vi "TreeItem.Property.Get.vi"(6 "Custom Device Path":string, 8 "error in (no error)":errorcluster, 9 "Default Value":variant, 10 "Property Name":string, 11 "Basenode":refnum<k24>) -> (0 "error out":errorcluster, 1 "Variant":variant, 2 "Found?":bool, 3 "Basenode":refnum<k24>)   [LabVIEW 2016, in "Advanced System Definition.lvlib"]
uses:
  SysDef API/Advanced System Definition.lvlib
  NationalInstruments.VeriStand.SystemStorage
  _Types/Property.DependentFile.ctl
  NationalInstruments.VeriStand
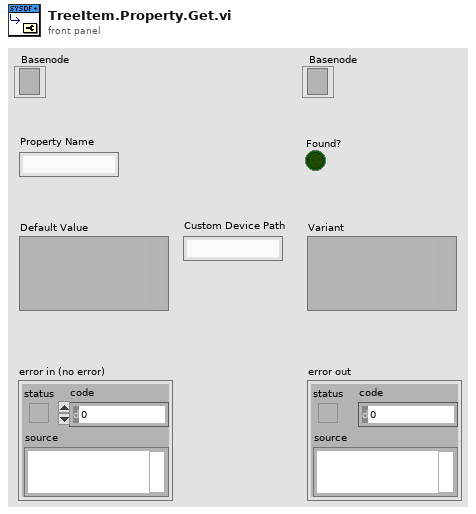
[diagram p1: front panel]
types:
  T1 = typedef "Advanced System Definition.lvlib/Property.DependentFile.ctl" = cluster{"Original Path":path, "Version":string, "RTDestination":path, "ForceDownload":bool, "SupportedTarget":string, "MD5":string}
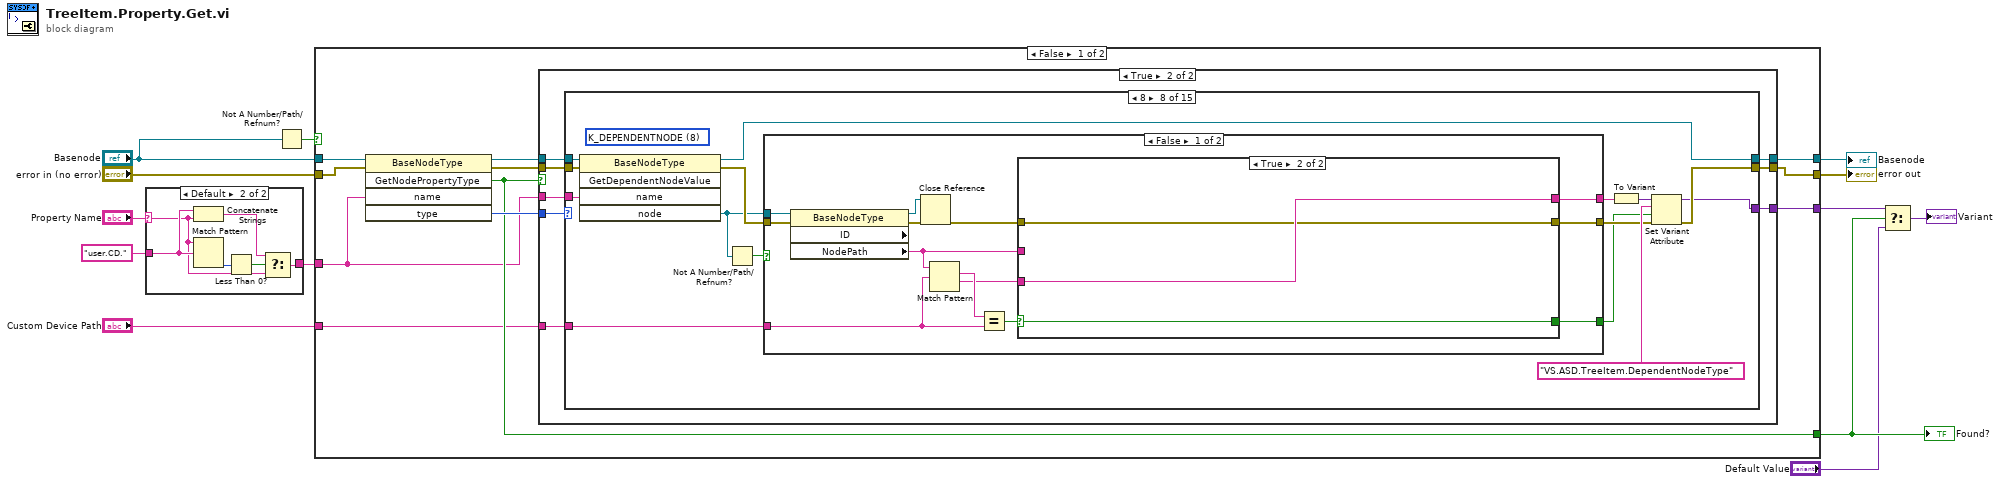
[diagram p0: block diagram]
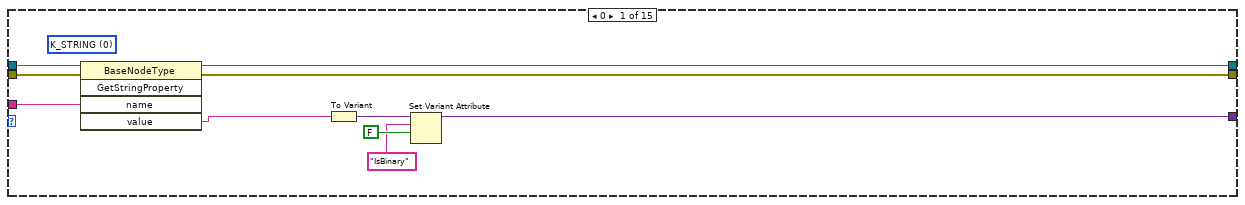
[diagram p4: hidden frame]
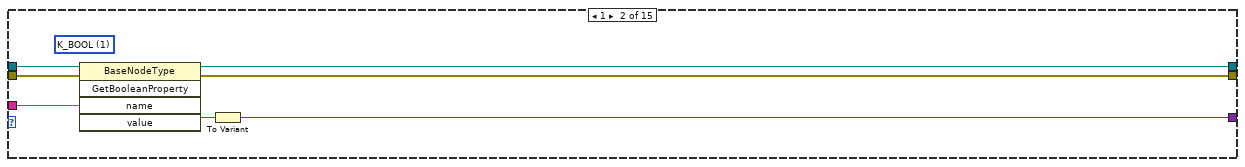
[diagram p5: hidden frame]
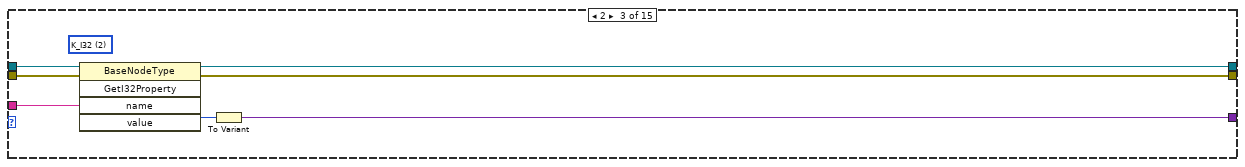
[diagram p6: hidden frame]
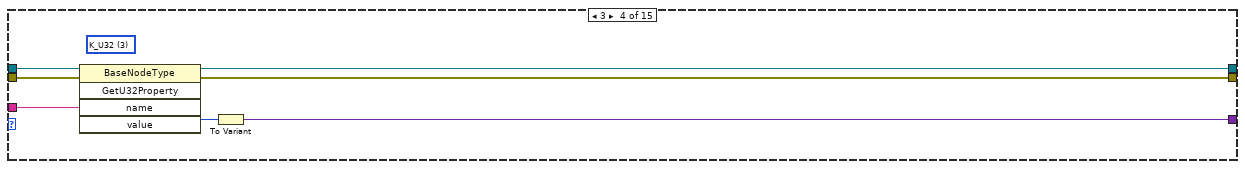
[diagram p7: hidden frame]
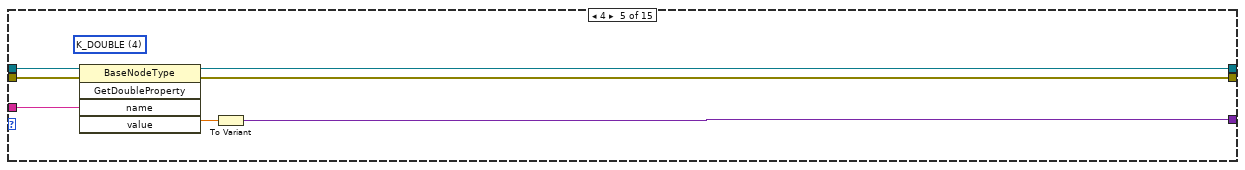
[diagram p8: hidden frame]
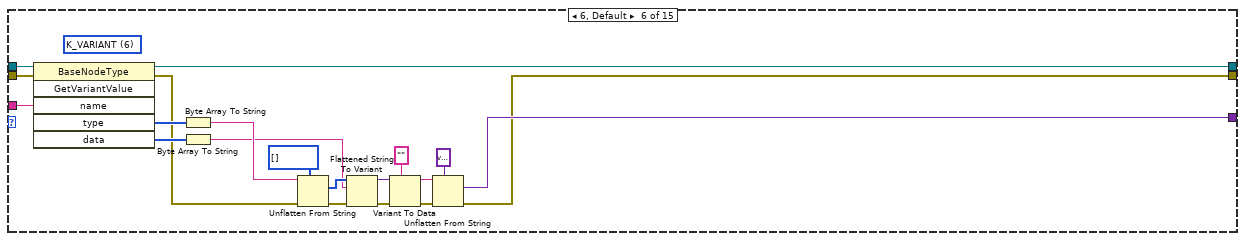
[diagram p9: hidden frame]
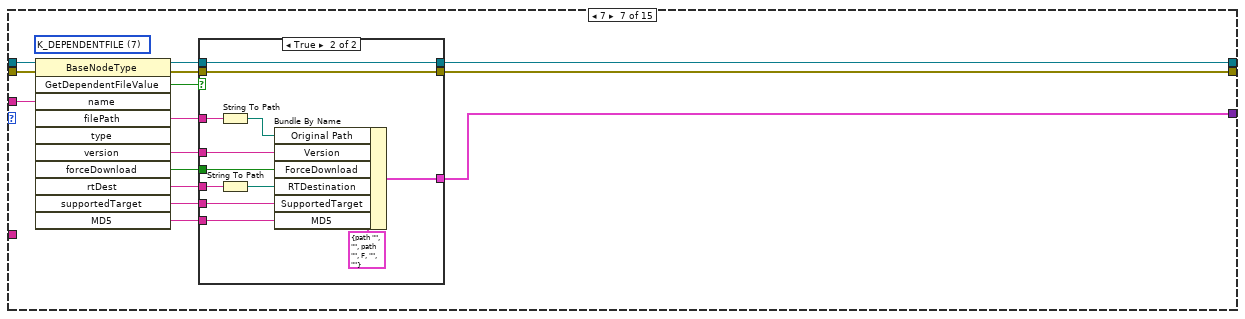
[diagram p10: hidden frame]
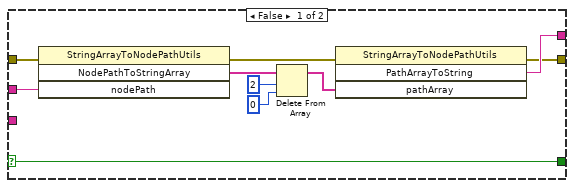
[diagram p12: hidden frame]
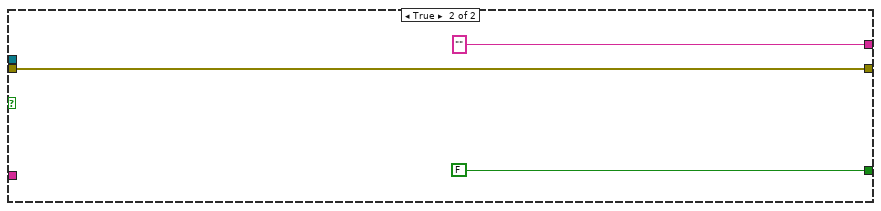
[diagram p13: hidden frame]
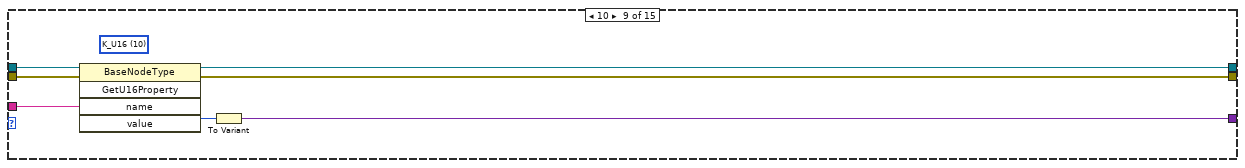
[diagram p14: hidden frame]
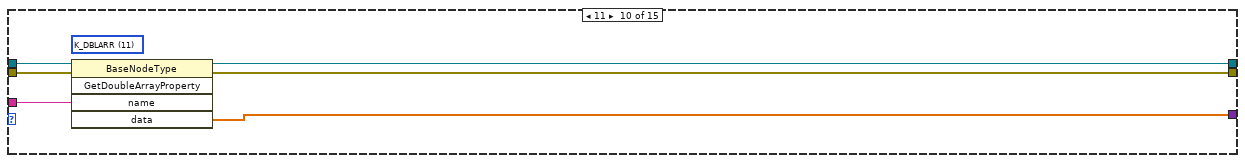
[diagram p15: hidden frame]
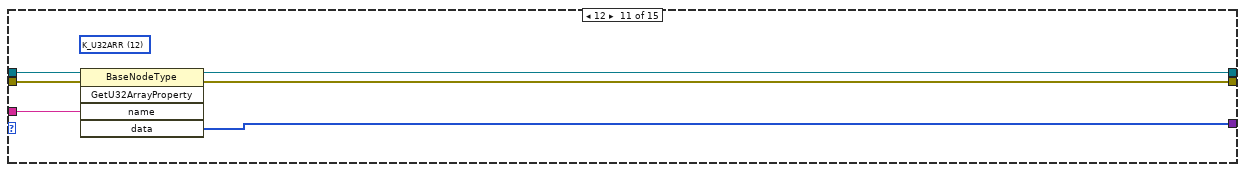
[diagram p16: hidden frame]
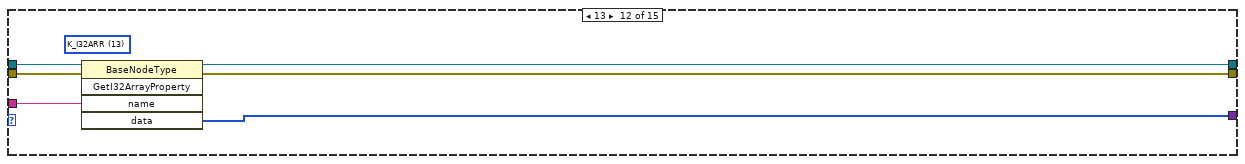
[diagram p17: hidden frame]
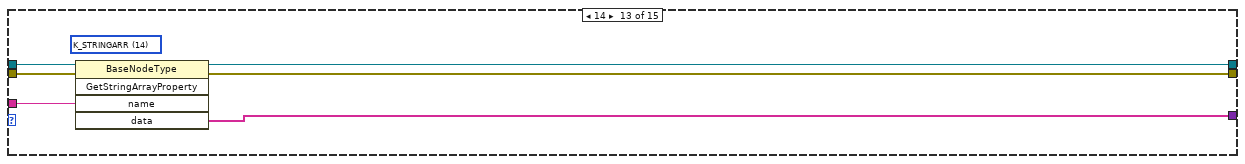
[diagram p18: hidden frame]
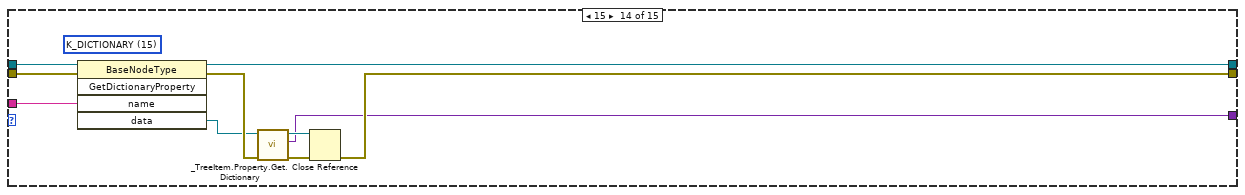
[diagram p19: hidden frame]
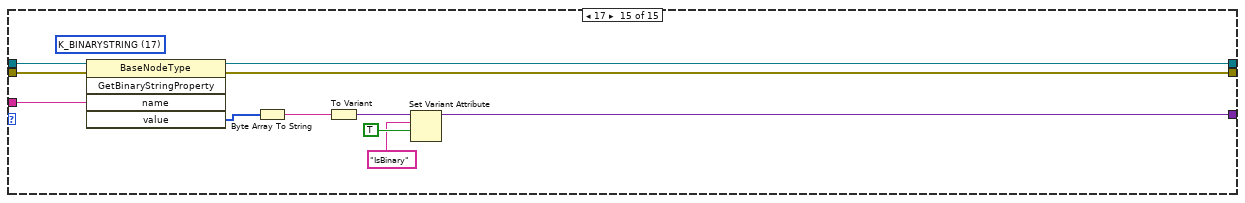
[diagram p20: hidden frame]
diagram:
  n1 = case shown="Default" "Property Name" {
    selector: "Property Name" -> [w14 w15]
    tunnel: "user.CD." ("regular expression") -> [_ w18]
    tunnel: [w14 w16] -> w3
    frame "Value Table" {
    }
    frame Default {
      n2 = Concatenate Strings(w18, w15) -> (w19:string)
      n3 = Match Pattern(string=w15, regular expression=w18) -> (offset past match=w20:i32)  [unwired: 1 in, 3 out]
      n4 = Less Than 0?(x=w20) -> (x < 0?=w17:bool)
      n5 = Select(t=w19, s=w17, f=w15) -> (s? t:f=w16:string)
    }
  }
  n6 = Not A Number/Path/Refnum?(number/path/refnum="Basenode") -> (NaN/Path/Refnum?=w13:bool)
  n7 = case shown="False" w13 {
    tunnel: w3 -> [w22 _]
    tunnel: "Basenode" -> [w31 w226]
    tunnel: "error in (no error)" -> [w30 w225]
    tunnel: [w26 _] -> w10
    tunnel: [w25 _] -> w9
    tunnel: [w24 w226] -> w6
    tunnel: [w23 w225] -> w5
    tunnel: "Custom Device Path" -> [w21 _]
    frame False {
      n8 = invoke class="BaseNodeType" method="GetNodePropertyType"(reference=w31, error in=w30, "name"=w22) -> (reference out=w27:refnum<k24>, error out=w29:errorcluster, "GetNodePropertyType"=w26:bool, "type"=w28:i32)  [unwired: 2 in, 1 out]
      n9 = case shown="True" w26 {
        tunnel: [w32 w41] -> w24
        tunnel: [w33 w40] -> w23
        tunnel: [_ w39] -> w25
        tunnel: w29 -> [w33 w38]
        tunnel: w28 -> [_ w37]
        tunnel: w27 -> [w32 w36]
        tunnel: w22 -> [_ w35]
        tunnel: w21 -> [_ w34]
        frame False {
        }
        frame True {
          n10 = case shown="8" w37 {
            tunnel: [w51 w58 w65 w72 w79 w99 w101 w140 w179 w185 w191 w197 w199 w212 w219] -> w41
            tunnel: w38 -> [w50 w57 w64 w71 w78 w98 w110 w143 w178 w184 w190 w196 w203 w213 w223]
            tunnel: [w49 w56 w63 w70 w77 w81 w102 w139 w177 w183 w189 w195 w202 w207 w220] -> w40
            tunnel: [w42 w54 w61 w68 w75 w82 w100 w138 w175 w182 w188 w194 w201 w205 w214] -> w39
            tunnel: w36 -> [w47 w53 w59 w66 w73 w97 w111 w142 w174 w180 w187 w193 w198 w211 w224]
            tunnel: w35 -> [w48 w52 w60 w67 w74 w96 w109 w141 w173 w181 w186 w192 w200 w204 w222]
            tunnel: w34 -> [_ _ _ _ _ _ _ w132 _ _ _ _ _ _ _]
            frame 0 {
              (unwired) 0 items=["K_STRING", "K_BOOL", "K_I32", "K_U32", "K_DOUBLE", "K_U64", "K_VARIANT", "K_DEPENDENTFILE", "K_DEPENDENTNODE", "K_DATASOURCENODE", "K_U16", "K_DBLARR", "K_U32ARR", "K_I32ARR", "K_STRINGARR", "K_DICTIONARY", "K_DICTIONARYARR"] ("type")
              n11 = invoke class="BaseNodeType" method="GetStringProperty"(reference=w47, error in=w50, "name"=w48) -> (reference out=w51:refnum<k24>, error out=w49:errorcluster, "value"=w43:string)  [unwired: 2 in, 2 out]
              n12 = To Variant(anything=w43) -> (Variant=w44:variant)
              n13 = Set Variant Attribute(Variant=w44, name="IsBinary", value=FALSE ("Set String as Binary")) -> (Variant out=w42:variant)  [unwired: 1 in, 2 out]
            }
            frame 1 {
              (unwired) 1 items=["K_STRING", "K_BOOL", "K_I32", "K_U32", "K_DOUBLE", "K_U64", "K_VARIANT", "K_DEPENDENTFILE", "K_DEPENDENTNODE", "K_DATASOURCENODE", "K_U16", "K_DBLARR", "K_U32ARR", "K_I32ARR", "K_STRINGARR", "K_DICTIONARY", "K_DICTIONARYARR"] ("type")
              n14 = invoke class="BaseNodeType" method="GetBooleanProperty"(reference=w53, error in=w57, "name"=w52) -> (reference out=w58:refnum<k24>, error out=w56:errorcluster, "value"=w55:bool)  [unwired: 2 in, 2 out]
              n15 = To Variant(anything=w55) -> (Variant=w54:variant)
            }
            frame 2 {
              (unwired) 2 items=["K_STRING", "K_BOOL", "K_I32", "K_U32", "K_DOUBLE", "K_U64", "K_VARIANT", "K_DEPENDENTFILE", "K_DEPENDENTNODE", "K_DATASOURCENODE", "K_U16", "K_DBLARR", "K_U32ARR", "K_I32ARR", "K_STRINGARR", "K_DICTIONARY", "K_DICTIONARYARR"] ("type")
              n16 = invoke class="BaseNodeType" method="GetI32Property"(reference=w59, error in=w64, "name"=w60) -> (reference out=w65:refnum<k24>, error out=w63:errorcluster, "value"=w62:i32)  [unwired: 2 in, 2 out]
              n17 = To Variant(anything=w62) -> (Variant=w61:variant)
            }
            frame 3 {
              (unwired) 3 items=["K_STRING", "K_BOOL", "K_I32", "K_U32", "K_DOUBLE", "K_U64", "K_VARIANT", "K_DEPENDENTFILE", "K_DEPENDENTNODE", "K_DATASOURCENODE", "K_U16", "K_DBLARR", "K_U32ARR", "K_I32ARR", "K_STRINGARR", "K_DICTIONARY", "K_DICTIONARYARR"] ("type")
              n18 = invoke class="BaseNodeType" method="GetU32Property"(reference=w66, error in=w71, "name"=w67) -> (reference out=w72:refnum<k24>, error out=w70:errorcluster, "value"=w69:u32)  [unwired: 2 in, 2 out]
              n19 = To Variant(anything=w69) -> (Variant=w68:variant)
            }
            frame 4 {
              (unwired) 4 items=["K_STRING", "K_BOOL", "K_I32", "K_U32", "K_DOUBLE", "K_U64", "K_VARIANT", "K_DEPENDENTFILE", "K_DEPENDENTNODE", "K_DATASOURCENODE", "K_U16", "K_DBLARR", "K_U32ARR", "K_I32ARR", "K_STRINGARR", "K_DICTIONARY", "K_DICTIONARYARR"] ("type")
              n20 = invoke class="BaseNodeType" method="GetDoubleProperty"(reference=w73, error in=w78, "name"=w74) -> (reference out=w79:refnum<k24>, error out=w77:errorcluster, "value"=w76:dbl)  [unwired: 2 in, 2 out]
              n21 = To Variant(anything=w76) -> (Variant=w75:variant)
            }
            frame 6, Default {
              (unwired) 6 items=["K_STRING", "K_BOOL", "K_I32", "K_U32", "K_DOUBLE", "K_U64", "K_VARIANT", "K_DEPENDENTFILE", "K_DEPENDENTNODE", "K_DATASOURCENODE", "K_U16", "K_DBLARR", "K_U32ARR", "K_I32ARR", "K_STRINGARR", "K_DICTIONARY", "K_DICTIONARYARR"] ("type")
              n22 = invoke class="BaseNodeType" method="GetVariantValue"(reference=w97, error in=w98, "name"=w96) -> (reference out=w99:refnum<k24>, error out=w80:errorcluster, "type"=w83:u8[], "data"=w84:u8[])  [unwired: 3 in, 2 out]
              n23 = Byte Array To String(unsigned byte array=w83) -> (string=w92:string)
              n24 = Byte Array To String(unsigned byte array=w84) -> (string=w91:string)
              n25 = Unflatten From String(type=i16[] [] ("type string"), binary string=w92, error in (no error)=w80) -> (value=w94:i16[], error out=w93:errorcluster)  [unwired: 2 in, 1 out]
              n26 = Flattened String To Variant(4:w93, 6:w91, 7:w94) -> (0:w87:errorcluster, 3:w90:variant)
              n27 = Variant To Data(error in=w87, type="", Variant=w90) -> (data=w88:string, error out=w86:errorcluster)
              n28 = Unflatten From String(type=variant ("variant"), binary string=w88, error in (no error)=w86) -> (value=w82:variant, error out=w81:errorcluster)  [unwired: 2 in, 1 out]
            }
            frame 7 {
              (unwired) 7 items=["K_STRING", "K_BOOL", "K_I32", "K_U32", "K_DOUBLE", "K_U64", "K_VARIANT", "K_DEPENDENTFILE", "K_DEPENDENTNODE", "K_DATASOURCENODE", "K_U16", "K_DBLARR", "K_U32ARR", "K_I32ARR", "K_STRINGARR", "K_DICTIONARY", "K_DICTIONARYARR"] ("type")
              n29 = invoke class="BaseNodeType" method="GetDependentFileValue"(reference=w111, error in=w110, "name"=w109) -> (reference out=w113:refnum<k24>, error out=w112:errorcluster, "GetDependentFileValue"=w114:bool, "filePath"=w108:string, "version"=w107:string, "forceDownload"=w105:bool, "rtDest"=w106:string, "supportedTarget"=w104:string, "MD5"=w103:string)  [unwired: 8 in, 2 out]
              n30 = case shown="True" w114 {
                tunnel: [w115 w119] -> w102
                tunnel: [w116 w125] -> w101
                tunnel: [_ w128] -> w100
                tunnel: w112 -> [w115 w119]
                tunnel: w113 -> [w116 w125]
                tunnel: w108 -> [_ w124]
                tunnel: w107 -> [_ w123]
                tunnel: w106 -> [_ w122]
                tunnel: w105 -> [_ w118]
                tunnel: w104 -> [_ w121]
                tunnel: w103 -> [_ w120]
                frame False {
                }
                frame True {
                  n31 = String To Path(string=w124) -> (path=w117:path)
                  n32 = String To Path(string=w122) -> (path=w126:path)
                  n33 = Bundle By Name(cluster=T1 {"Original Path"=path "", "Version"="", "RTDestination"=path "", "ForceDownload"=FALSE, "SupportedTarget"="", "MD5"=""} ("OptionalInfo"), "Original Path"=w117, "Version"=w123, "ForceDownload"=w118, "RTDestination"=w126, "SupportedTarget"=w121, "MD5"=w120) -> (w128:T1)
                }
              }
            }
            frame 8 {
              (unwired) 8 items=["K_STRING", "K_BOOL", "K_I32", "K_U32", "K_DOUBLE", "K_U64", "K_VARIANT", "K_DEPENDENTFILE", "K_DEPENDENTNODE", "K_DATASOURCENODE", "K_U16", "K_DBLARR", "K_U32ARR", "K_I32ARR", "K_STRINGARR", "K_DICTIONARY", "K_DICTIONARYARR"] ("type")
              n34 = invoke class="BaseNodeType" method="GetDependentNodeValue"(reference=w142, error in=w143, "name"=w141) -> (reference out=w140:refnum<k24>, error out=w134:errorcluster, "node"=w133:refnum<k24>)  [unwired: 2 in, 2 out]
              n35 = Not A Number/Path/Refnum?(number/path/refnum=w133) -> (NaN/Path/Refnum?=w135:bool)
              n36 = case shown="False" w135 {
                tunnel: w134 -> [w153 w172]
                tunnel: [w146 w172] -> w130
                tunnel: w133 -> [w154 _]
                tunnel: w132 -> [w151 _]
                tunnel: [w145 "" ("NodePath")] -> w131
                tunnel: [w144 FALSE] -> w129
                frame False {
                  n37 = property class="BaseNodeType" props=["ID", "NodePath"](reference=w154, error in=w153) -> (reference out=w155:refnum<k24>, error out=w156:errorcluster, "NodePath"=w148:string)  [unwired: 1 out]
                  n38 = Close Reference(reference=w155, error in (no error)=w156) -> (error out=w147:errorcluster)
                  n39 = Match Pattern(string=w148, regular expression=w151) -> (match substring=w152:string, after substring=w149:string)  [unwired: 1 in, 2 out]
                  n40 = Equal?(x=w152, y=w151) -> (x = y?=w150:bool)
                  n41 = case shown="True" w150 {
                    selector: w150 -> [w166 w168]
                    tunnel: [w166 w168] -> w144
                    tunnel: [w158 w169] -> w145
                    tunnel: w149 -> [_ w169]
                    tunnel: w148 -> [w165 _]
                    tunnel: w147 -> [w159 w167]
                    tunnel: [w157 w167] -> w146
                    frame False {
                      n42 = invoke class="StringArrayToNodePathUtils" method="NodePathToStringArray"(error in=w159, "nodePath"=w165) -> (error out=w160:errorcluster, "NodePathToStringArray"=w164:string[])  [unwired: 2 in, 2 out]
                      n43 = Delete From Array(array=w164, length=2, index=0) -> (array with subset deleted=w161:string[])  [unwired: 1 out]
                      n44 = invoke class="StringArrayToNodePathUtils" method="PathArrayToString"(error in=w160, "pathArray"=w161) -> (error out=w157:errorcluster, "PathArrayToString"=w158:string)  [unwired: 2 in, 2 out]
                    }
                    frame True {
                    }
                  }
                }
                frame True {
                }
              }
              n45 = To Variant(anything=w131) -> (Variant=w137:variant)
              n46 = Set Variant Attribute(Variant=w137, name="VS.ASD.TreeItem.DependentNodeType", value=w129, error in=w130) -> (Variant out=w138:variant, error out=w139:errorcluster)  [unwired: 1 out]
            }
            frame 10 {
              (unwired) 10 items=["K_STRING", "K_BOOL", "K_I32", "K_U32", "K_DOUBLE", "K_U64", "K_VARIANT", "K_DEPENDENTFILE", "K_DEPENDENTNODE", "K_DATASOURCENODE", "K_U16", "K_DBLARR", "K_U32ARR", "K_I32ARR", "K_STRINGARR", "K_DICTIONARY", "K_DICTIONARYARR"] ("type")
              n47 = invoke class="BaseNodeType" method="GetU16Property"(reference=w174, error in=w178, "name"=w173) -> (reference out=w179:refnum<k24>, error out=w177:errorcluster, "value"=w176:u16)  [unwired: 2 in, 2 out]
              n48 = To Variant(anything=w176) -> (Variant=w175:variant)
            }
            frame 11 {
              (unwired) 11 items=["K_STRING", "K_BOOL", "K_I32", "K_U32", "K_DOUBLE", "K_U64", "K_VARIANT", "K_DEPENDENTFILE", "K_DEPENDENTNODE", "K_DATASOURCENODE", "K_U16", "K_DBLARR", "K_U32ARR", "K_I32ARR", "K_STRINGARR", "K_DICTIONARY", "K_DICTIONARYARR"] ("type")
              n49 = invoke class="BaseNodeType" method="GetDoubleArrayProperty"(reference=w180, error in=w184, "name"=w181) -> (reference out=w185:refnum<k24>, error out=w183:errorcluster, "data"=w182:dbl[])  [unwired: 2 in, 2 out]
            }
            frame 12 {
              (unwired) 12 items=["K_STRING", "K_BOOL", "K_I32", "K_U32", "K_DOUBLE", "K_U64", "K_VARIANT", "K_DEPENDENTFILE", "K_DEPENDENTNODE", "K_DATASOURCENODE", "K_U16", "K_DBLARR", "K_U32ARR", "K_I32ARR", "K_STRINGARR", "K_DICTIONARY", "K_DICTIONARYARR"] ("type")
              n50 = invoke class="BaseNodeType" method="GetU32ArrayProperty"(reference=w187, error in=w190, "name"=w186) -> (reference out=w191:refnum<k24>, error out=w189:errorcluster, "data"=w188:u32[])  [unwired: 2 in, 2 out]
            }
            frame 13 {
              (unwired) 13 items=["K_STRING", "K_BOOL", "K_I32", "K_U32", "K_DOUBLE", "K_U64", "K_VARIANT", "K_DEPENDENTFILE", "K_DEPENDENTNODE", "K_DATASOURCENODE", "K_U16", "K_DBLARR", "K_U32ARR", "K_I32ARR", "K_STRINGARR", "K_DICTIONARY", "K_DICTIONARYARR"] ("type")
              n51 = invoke class="BaseNodeType" method="GetI32ArrayProperty"(reference=w193, error in=w196, "name"=w192) -> (reference out=w197:refnum<k24>, error out=w195:errorcluster, "data"=w194:i32[])  [unwired: 2 in, 2 out]
            }
            frame 14 {
              (unwired) 14 items=["K_STRING", "K_BOOL", "K_I32", "K_U32", "K_DOUBLE", "K_U64", "K_VARIANT", "K_DEPENDENTFILE", "K_DEPENDENTNODE", "K_DATASOURCENODE", "K_U16", "K_DBLARR", "K_U32ARR", "K_I32ARR", "K_STRINGARR", "K_DICTIONARY", "K_DICTIONARYARR"] ("type")
              n52 = invoke class="BaseNodeType" method="GetStringArrayProperty"(reference=w198, error in=w203, "name"=w200) -> (reference out=w199:refnum<k24>, error out=w202:errorcluster, "data"=w201:string[])  [unwired: 2 in, 2 out]
            }
            frame 15 {
              (unwired) 15 items=["K_STRING", "K_BOOL", "K_I32", "K_U32", "K_DOUBLE", "K_U64", "K_VARIANT", "K_DEPENDENTFILE", "K_DEPENDENTNODE", "K_DATASOURCENODE", "K_U16", "K_DBLARR", "K_U32ARR", "K_I32ARR", "K_STRINGARR", "K_DICTIONARY", "K_DICTIONARYARR"] ("type")
              n53 = invoke class="BaseNodeType" method="GetDictionaryProperty"(reference=w211, error in=w213, "name"=w204) -> (reference out=w212:refnum<k24>, error out=w210:errorcluster, "data"=w209:refnum<k24>)  [unwired: 2 in, 2 out]
              n54 = call "_TreeItem.Property.Get.Dictionary.vi"("error in (no error)"=w210, "DictionaryProperty"=w209) -> ("error out"=w208:errorcluster, "Dictionary Variant"=w205:variant, "DictionaryProperty out"=w206:refnum<k24>)  [unwired: 7 in]
              n55 = Close Reference(reference=w206, error in (no error)=w208) -> (error out=w207:errorcluster)
            }
            frame 17 {
              (unwired) 17 items=["K_STRING", "K_BOOL", "K_I32", "K_U32", "K_DOUBLE", "K_U64", "K_VARIANT", "K_DEPENDENTFILE", "K_DEPENDENTNODE", "K_DATASOURCENODE", "K_U16", "K_DBLARR", "K_U32ARR", "K_I32ARR", "K_STRINGARR", "K_DICTIONARY", "K_DICTIONARYARR", "K_BINARYSTRING"] ("type")
              n56 = invoke class="BaseNodeType" method="GetBinaryStringProperty"(reference=w224, error in=w223, "name"=w222) -> (reference out=w219:refnum<k24>, error out=w220:errorcluster, "value"=w221:u8[])  [unwired: 2 in, 2 out]
              n57 = Byte Array To String(unsigned byte array=w221) -> (string=w215:string)
              n58 = To Variant(anything=w215) -> (Variant=w216:variant)
              n59 = Set Variant Attribute(Variant=w216, name="IsBinary", value=TRUE ("Set String as Binary")) -> (Variant out=w214:variant)  [unwired: 1 in, 2 out]
            }
          }
        }
      }
    }
    frame True {
    }
  }
  "Basenode" <- w6
  "Found?" <- w10
  "error out" <- w5
  n60 = Select(t=w9, s=w10, f="Default Value") -> (s? t:f=→"Variant":variant)
